vi "Gravar.vi"(8 "error in (no error)":errorcluster, 11 "SP Dados In":T1={"Condutor"={"Pc (N/m)"=0.0, "Mod.Young (N/m²)"=0.0, "Dil.Term.c (m/°C)"=0.0, "Área  (m²)"=0.0, "Tração EDS (N)"=0.0, "Tração Torig(N)"=0.0, "Tração Talta (N)"=0.0}, "Suporte"={"Ps (N/m)"=0.0, "Es (N/m²)"=0.0, "DTc (1/°C)"=0.0, "Área sup (m²)"=0.0, "Tração EDS sup (N)"=0.0, "Tração AT sup (N)"=0.0, "Flecha sup AT (m)"=0.0}, "Projeto"={"Temp. EDS (°C)"=0.0, "Lim.original (°C)"=0.0, "Lim.extend. (°C)"=0.0, "N. cabo/fase"=1.0}, "Vetor de dados"={"Coor.X.esp"=[], "Coor.Y.Esp."=[], "Sub.vao X"=[], "Sub.vao Y"=[], "CoordY.sup"=[], "CoordX.sup"=[]}, "Subvão"={"N. Esp."=0.0, "F.lim (m)"=0.0, "Ext.calc"=0.0, "Ext.definido"=0.0, "Comp.cabo"=0.0, "Ext.55%"=0.0, "Tração sub\nAT (N)"=0.0, "Ext.sel."=0.0, "Flecha lim.\ncalc (m)"=0.0}, "Vão"={"Extensão (m)"=0.0, "Desnivel (m)"=0.0, "Ext.Lim sub (m)"=0.0, "Flecha à 60 °C"=0.0}} {"Projeto"."N. cabo/fase" min=1.0 max=8.0 step=1.0 format="%#_1f"}) -> (0 "error out":errorcluster, 3 "SP Dados Out":T1={"Condutor"={"Pc (N/m)"=0.0, "Mod.Young (N/m²)"=0.0, "Dil.Term.c (m/°C)"=0.0, "Área  (m²)"=0.0, "Tração EDS (N)"=0.0, "Tração Torig(N)"=0.0, "Tração Talta (N)"=0.0}, "Suporte"={"Ps (N/m)"=0.0, "Es (N/m²)"=0.0, "DTc (1/°C)"=0.0, "Área sup (m²)"=0.0, "Tração EDS sup (N)"=0.0, "Tração AT sup (N)"=0.0, "Flecha sup AT (m)"=0.0}, "Projeto"={"Temp. EDS (°C)"=0.0, "Lim.original (°C)"=0.0, "Lim.extend. (°C)"=0.0, "N. cabo/fase"=1.0}, "Vetor de dados"={"Coor.X.esp"=[], "Coor.Y.Esp."=[], "Sub.vao X"=[], "Sub.vao Y"=[], "CoordY.sup"=[], "CoordX.sup"=[]}, "Subvão"={"N. Esp."=0.0, "F.lim (m)"=0.0, "Ext.calc"=0.0, "Ext.definido"=0.0, "Comp.cabo"=0.0, "Ext.55%"=0.0, "Tração sub\nAT (N)"=0.0, "Ext.sel."=0.0, "Flecha lim.\ncalc (m)"=0.0}, "Vão"={"Extensão (m)"=0.0, "Desnivel (m)"=0.0, "Ext.Lim sub (m)"=0.0, "Flecha à 60 °C"=0.0}} {"Projeto"."N. cabo/fase" min=1.0 max=8.0 step=1.0 format="%#_1f"})   [LabVIEW 2020]
uses:
  controles/SP data.ctl
  <vilib>/Utility/file.llb/Write Delimited Spreadsheet (string).vi
  <vilib>/Utility/file.llb/Write Delimited Spreadsheet (DBL).vi
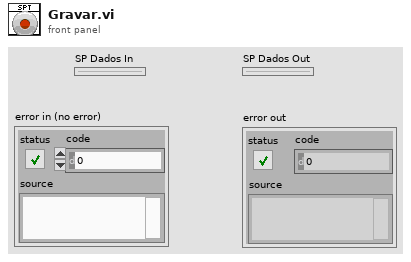
[diagram p1: front panel]
types:
  T1 = typedef "SP data.ctl" = cluster{"Condutor":cluster{"Pc (N/m)":dbl, "Mod.Young (N/m²)":dbl, "Dil.Term.c (m/°C)":dbl, "Área  (m²)":dbl, "Tração EDS (N)":dbl, "Tração Torig(N)":dbl, "Tração Talta (N)":dbl}, "Suporte":cluster{"Ps (N/m)":dbl, "Es (N/m²)":dbl, "DTc (1/°C)":dbl, "Área sup (m²)":dbl, "Tração EDS sup (N)":dbl, "Tração AT sup (N)":dbl, "Flecha sup AT (m)":dbl}, "Projeto":cluster{"Temp. EDS (°C)":dbl, "Lim.original (°C)":dbl, "Lim.extend. (°C)":dbl, "N. cabo/fase":dbl}, "Vetor de dados":cluster{"Coor.X.esp":dbl[], "Coor.Y.Esp.":dbl[], "Sub.vao X":dbl[], "Sub.vao Y":dbl[], "CoordY.sup":dbl[], "CoordX.sup":dbl[]}, "Subvão":cluster{"N. Esp.":dbl, "F.lim (m)":dbl, "Ext.calc":dbl, "Ext.definido":dbl, "Comp.cabo":dbl, "Ext.55%":dbl, "Tração sub\nAT (N)":dbl, "Ext.sel.":dbl, "Flecha lim.\ncalc (m)":dbl}, "Vão":cluster{"Extensão (m)":dbl, "Desnivel (m)":dbl, "Ext.Lim sub (m)":dbl, "Flecha à 60 °C":dbl}}
  T2 = cluster{"Pc (N/m)":dbl, "Mod.Young (N/m²)":dbl, "Dil.Term.c (m/°C)":dbl, "Área  (m²)":dbl, "Tração EDS (N)":dbl, "Tração Torig(N)":dbl, "Tração Talta (N)":dbl}
  T3 = cluster{"Ps (N/m)":dbl, "Es (N/m²)":dbl, "DTc (1/°C)":dbl, "Área sup (m²)":dbl, "Tração EDS sup (N)":dbl, "Tração AT sup (N)":dbl, "Flecha sup AT (m)":dbl}
  T4 = cluster{"Extensão (m)":dbl, "Desnivel (m)":dbl, "Ext.Lim sub (m)":dbl, "Flecha à 60 °C":dbl}
  T5 = cluster{"Temp. EDS (°C)":dbl, "Lim.original (°C)":dbl, "Lim.extend. (°C)":dbl, "N. cabo/fase":dbl}
  T6 = cluster{"N. Esp.":dbl, "F.lim (m)":dbl, "Ext.calc":dbl, "Ext.definido":dbl, "Comp.cabo":dbl, "Ext.55%":dbl, "Tração sub\nAT (N)":dbl, "Ext.sel.":dbl, "Flecha lim.\ncalc (m)":dbl}
  T7 = cluster{"Coor.X.esp":dbl[], "Coor.Y.Esp.":dbl[], "Sub.vao X":dbl[], "Sub.vao Y":dbl[], "CoordY.sup":dbl[], "CoordX.sup":dbl[]}
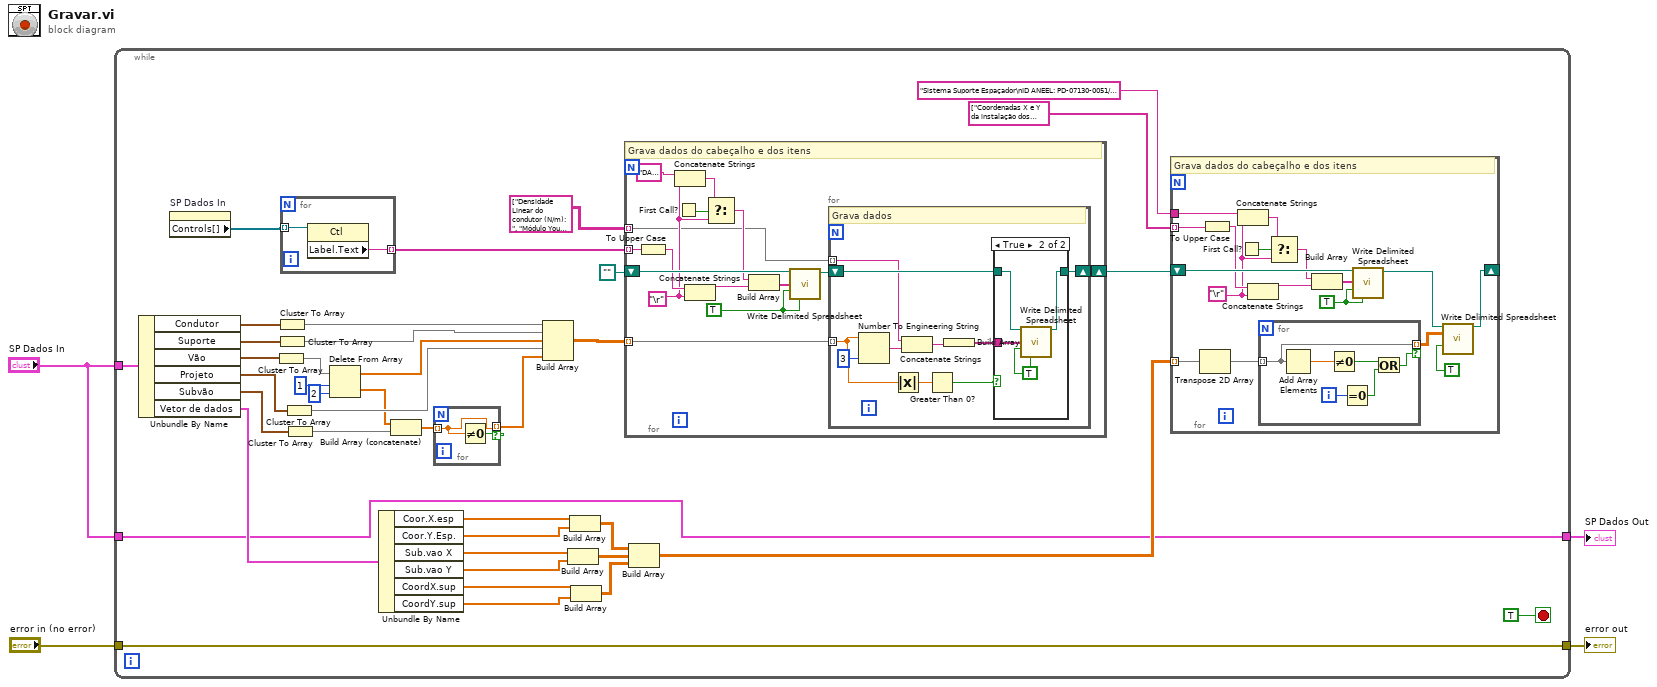
[diagram p0: block diagram]
diagram:
  n1 = while {
    tunnel: "SP Dados In" -> [w17]
    tunnel: "error in (no error)" -> [w16]
    tunnel: [w16] -> w3
    tunnel: "SP Dados In" -> [w15]
    tunnel: [w15] -> w1
    stop <- TRUE stop-if-true
    n2 = Unbundle By Name(w17) -> ("Condutor"=w43:T2, "Suporte"=w42:T3, "Vão"=w41:T4, "Projeto"=w34:T5, "Subvão"=w31:T6, "Vetor de dados"=w30:T7)
    n3 = property on="SP Dados In" class="Clust (strict)"() -> ("Controls[]"=w35:refnum<vi>[])  [unwired: 2 in, 2 out]
    n4 = Cluster To Array(cluster=w41) -> (array=w12:dbl[])
    n5 = Cluster To Array(cluster=w43) -> (array=w40:dbl[])
    n6 = Cluster To Array(cluster=w42) -> (array=w39:dbl[])
    n7 = for {
      tunnel: w35 -> [w100] mode=indexing
      tunnel: [w99] -> w37 mode=indexing
      n8 = property class="Ctl"(reference=w100) -> ("Label.Text"=w99:string)  [unwired: 1 in, 2 out]
    }
    n9 = Cluster To Array(cluster=w34) -> (array=w38:dbl[])
    n10 = Cluster To Array(cluster=w31) -> (array=w33:dbl[])
    n11 = Delete From Array(array=w12, length=1, index=2) -> (deleted portion=w8:dbl[], array with subset deleted=w9:dbl[])
    n12 = Unbundle By Name(w30) -> ("Coor.X.esp"=w29:dbl[], "Coor.Y.Esp."=w28:dbl[], "Sub.vao X"=w27:dbl[], "Sub.vao Y"=w26:dbl[], "CoordX.sup"=w25:dbl[], "CoordY.sup"=w24:dbl[])
    n13 = Build Array (concatenate)(w8, w33) -> (w7:dbl[])
    n14 = for {
      tunnel: w7 -> [w45] mode=indexing
      tunnel: [w45] -> w6 mode=indexing if=w44
      n15 = Not Equal To 0?(x=w45) -> (x != 0?=w44:bool)
    }
    n16 = Build Array(w40, w39, w9, w38, w6) -> (w36:dbl[][])
    n17 = Build Array(w27, w26) -> (w22:dbl[][])
    n18 = Build Array(w29, w28) -> (w23:dbl[][])
    n19 = Build Array(w25, w24) -> (w21:dbl[][])
    n20 = for {
      tunnel: w36 -> [w69] mode=indexing
      tunnel: w37 -> [w80] mode=indexing
      tunnel: string[][] [["Densidade Linear do condutor (N/m): ", "Módulo Young Condutor (N/m²): ", "Coeficiente de dilatação condutor (1/°C): ", "Seção transversal do condutor (mm²): ", "Tração EDS condutor c/ e s/ cabo suporte(N): ", "Tração do condutor Tm nominal s/ cabo suporte (°C): ", "Tração do condutor Tm ampliada s/ cabo suporte (°C): "], ["Densidade Linear do suporte (N/m): ", "Módulo Young Suporte (N/m²): ", "Coeficiente de dilatação suporte (1/°C): ", "Seção transversal do suporte (mm²): ", "Tração suporte à temp. EDS (N): ", "Tração suporte à temp. extendida (N): ", "Flecha Temperatura Estendida (m): "], ["Extensão do vão (m): ", "Desnível apoios (m): ", "Flecha a temperatura nominal de projeto (°C): ", "", "", "", ""], ["Temperatura EDS (°C)", "Temperatura limite original (°C)", "Temperatura limite estendida (°C)", "Número de cabos por fase: ", "", "", ""], ["Extensão do subvão limite (m)", "Número de espaçadores calculado: ", "Extensão limite calculada (m): ", "Extensão do subvão calculada (m): ", "Extensão do subvão calculada 55% (m): ", "Tração condutor temp max. (kN): ", "Extensão limite subvão sugerido (m): "]] -> [w70] mode=indexing
      shift-right: [w83] -> w18
      shift-left: path "" -> [w82]
      w71 = "\r"
      w79 = TRUE ("append to file? (new file:F)")
      # "Grava dados do cabeçalho e dos itens"
      n21 = To Upper Case(1:w80) -> (0:w76:string)
      n22 = First Call?() -> (First Call?: T/F=w75:bool)
      n23 = Concatenate Strings("DADOS DO PROGRAMA \nSPACER POSITION" ("concatenated string"), w71) -> (w72:string)
      n24 = Concatenate Strings(w76, w71) -> (w78:string)
      n25 = Select(t=w72, s=w75, f=w71) -> (s? t:f=w74:string)
      n26 = Build Array(w74, w78) -> (w77:string[])
      n27 = call-poly <vilib>:"Write Delimited Spreadsheet.vi"("file path (dialog if empty)"=w82, "1D data"=w77, "append to file? (new file:F)"=w79, "transpose? (no:F)"=w79) -> ("new file path (Not A Path if cancelled)"=w81:path)  [unwired: 10 in, 1 out]
      n28 = for {
        tunnel: w69 -> [w88] mode=indexing
        shift-right: [w90] -> w83
        shift-left: w81 -> [w89]
        tunnel: w70 -> [w84] mode=indexing
        # "Grava dados"
        n29 = Number To Engineering String(2:i16 3 ("precision (6)"), 4:w88) -> (0:w91:string)  [unwired: 2 in]
        n30 = Absolute Value(x=w88) -> (abs(x)=w87:dbl)
        n31 = Concatenate Strings(w84, w91) -> (w86:string)
        n32 = Greater Than 0?(x=w87) -> (x > 0?=w85:bool)
        n33 = Build Array(w86) -> (w93:string[])
        n34 = case shown="True" w85 {
          tunnel: w93 -> [_ w98]
          tunnel: [w94 w97] -> w90
          tunnel: w89 -> [w94 w96]
          frame False {
          }
          frame True {
            w95 = TRUE ("append to file? (new file:F)")
            n35 = call-poly <vilib>:"Write Delimited Spreadsheet.vi"("file path (dialog if empty)"=w96, "1D data"=w98, "append to file? (new file:F)"=w95, "transpose? (no:F)"=w95) -> ("new file path (Not A Path if cancelled)"=w97:path)  [unwired: 10 in, 1 out]
          }
        }
      }
    }
    n36 = Build Array(w23, w22, w21) -> (w19:dbl[][][])
    n37 = for {
      tunnel: w19 -> [w48] mode=indexing
      tunnel: string[] ["Coordenadas X e Y da instalação dos espaçadores (m)", "Coordenadas X e Y dos subvãos de condutores (m)", "Coordenadas X e Y do cabo suporte (m)"] -> [w49] mode=indexing
      shift-right: [w62] -> _
      shift-left: w18 -> [w61]
      tunnel: "Sistema Suporte Espaçador\nID ANEEL: PD-07130-0051/2020\nDados das Curvas\n" ("concatenated string") -> [w46]
      w52 = "\r"
      w59 = TRUE ("append to file? (new file:F)")
      # "Grava dados do cabeçalho e dos itens"
      n38 = Transpose 2D Array(2D array=w48) -> (transposed array=w47:dbl[][])
      n39 = To Upper Case(1:w49) -> (0:w56:string)
      n40 = First Call?() -> (First Call?: T/F=w55:bool)
      n41 = Concatenate Strings(w46, w52) -> (w53:string)
      n42 = Concatenate Strings(w56, w52) -> (w58:string)
      n43 = for {
        tunnel: w47 -> [w67] mode=indexing
        tunnel: [w67] -> w51 mode=indexing if=w65
        i -> [w66]
        n44 = Add Array Elements(numeric array=w67) -> (sum=w68:dbl)
        n45 = Not Equal To 0?(x=w68) -> (x != 0?=w64:bool)
        n46 = Equal To 0?(x=w66) -> (x = 0?=w63:bool)
        n47 = Or(x=w64, y=w63) -> (x .or. y?=w65:bool)
      }
      n48 = Select(t=w53, s=w55, f=w52) -> (s? t:f=w54:string)
      n49 = Build Array(w54, w58) -> (w57:string[])
      n50 = call-poly <vilib>:"Write Delimited Spreadsheet.vi"("file path (dialog if empty)"=w61, "1D data"=w57, "append to file? (new file:F)"=w59, "transpose? (no:F)"=w59) -> ("new file path (Not A Path if cancelled)"=w60:path)  [unwired: 10 in, 1 out]
      n51 = call-poly <vilib>:"Write Delimited Spreadsheet.vi"("file path (dialog if empty)"=w60, "2D data"=w51, "append to file? (new file:F)"=TRUE) -> ("new file path (Not A Path if cancelled)"=w62:path)  [unwired: 11 in, 1 out]
    }
  }
  "SP Dados Out" <- w1
  "error out" <- w3
